vi "Remove From Array If Not Corrupt.vi"(9 "Score":i32, 10 "Expected Char":string, 11 "Array in":string[](array[string])) -> (2 "Score":i32, 3 "Array out":string[](array[string]))   [LabVIEW 2019, in "Day 10.lvlib"]
uses:
  Day 10.lvlib
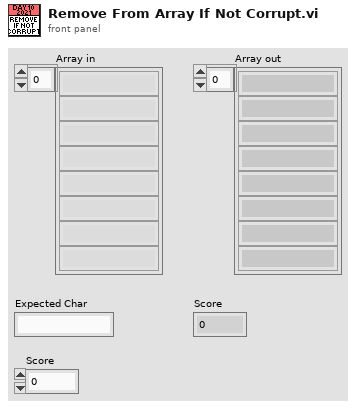
[diagram p1: front panel]
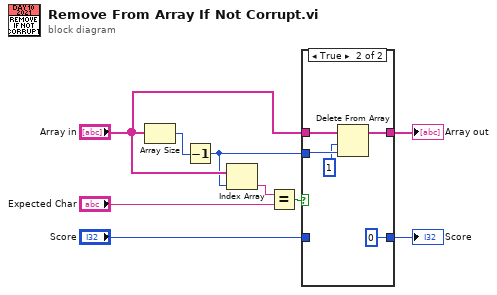
[diagram p0: block diagram]
diagram:
  n1 = Array Size(array="Array in") -> (size(s)=w2:i32)
  n2 = Decrement(x=w2) -> (x-1=w1:i32)
  n3 = Index Array(array="Array in", index=w1) -> (element=w3:string)
  n4 = Equal?(x=w3, y="Expected Char") -> (x = y?=w7:bool)
  n5 = case shown="True" w7 {
    tunnel: "Array in" -> [w11 w16]
    tunnel: w1 -> [_ w15]
    tunnel: [w11 w13] -> w6
    tunnel: [w10 0] -> w8
    tunnel: "Score" -> [w10 _]
    frame False {
    }
    frame True {
      n6 = Delete From Array(array=w16, length=1, index=w15) -> (array with subset deleted=w13:string[])  [unwired: 1 out]
    }
  }
  "Score" <- w8
  "Array out" <- w6
